vi "Pause.vi"(8 "error in":errorcluster, 9 "timeout (-1)":i32=-1, 11 "Standard Engine in":refnum<class "synchronous engine runtime.lvclass">) -> (0 "error out":errorcluster, 3 "Standard Engine out":refnum<class "synchronous engine runtime.lvclass">)   [LabVIEW 2013, in "synchronous engine runtime.lvclass"]
uses:
  synchronous engine runtime.lvclass
  Commands.ctl
  synchronous engine runtime.lvclass/synchronous engine runtime.ctl
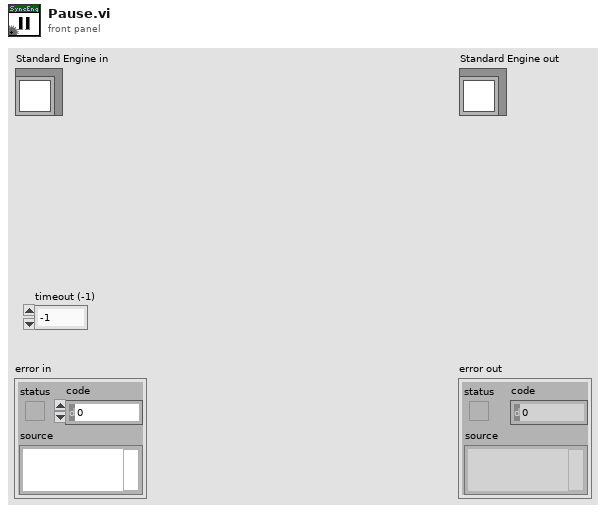
[diagram p1: front panel]
types:
  T1 = typedef "synchronous engine runtime.lvclass/Commands.ctl" = enum16{"Start", "Pause", "Safe State", "Normal", "Stop", "Shutdown"}
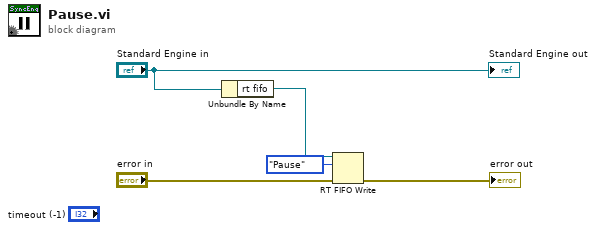
[diagram p0: block diagram]
diagram:
  n1 = Unbundle By Name("Standard Engine in") -> ("rt fifo"=w5:refnum<k33>)
  n2 = RT FIFO Write(0:w5, 1:Commands."Pause" ("element"), 3:"error in") -> (11:→"error out":errorcluster)  [unwired: 2 in, 3 out]
  "Standard Engine out" <- "Standard Engine in"
